vi "Number of Periods.vi"(7 "Read Value? (F)":bool, 8 "error in (no error)":errorcluster, 10 "Number of Periods (1)":u16=1 max=2000 step=1, 11 "VISA resource name":refnum<visa-resource-name>) -> (0 "error out":errorcluster, 2 "Number of Periods":u16=1, 3 "VISA resource name out":refnum<visa-resource-name>)   [LabVIEW 2013, in "SRS SR400.lvlib"]
doc: "<B>NP { m }</B>\n\nIf m is absent, the NP command returns the programmed number of periods in a scan (N PERIODS). If m is included, the number of periods is set to the value m. The parameter m must be an integer from 1 to 2000. Changing the number of periods during a scan is allowed. If the new value exceeds the current scan position, then the scan will continue to the new number of periods. If the new value is lower than the current scan position, then the scan ends at the next end of count period."
uses:
  <instrlib>/SRS SR400/SRS SR400.lvlib
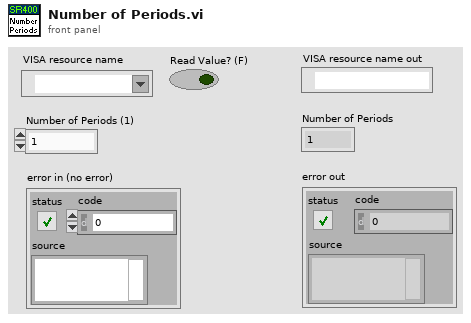
[diagram p1: front panel]
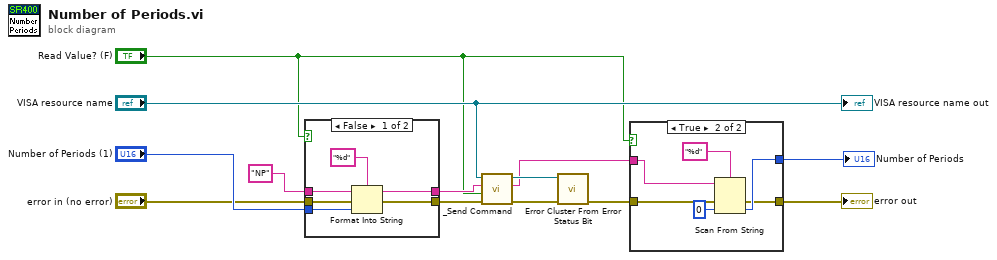
[diagram p0: block diagram]
diagram:
  n1 = case shown="False" "Read Value? (F)" {
    tunnel: "Number of Periods (1)" -> [w19 _]
    tunnel: "error in (no error)" -> [w18 w20]
    tunnel: "NP" ("command") -> [w16 w21]
    tunnel: [w15 w21] -> w10
    tunnel: [w14 w20] -> w9
    frame False {
      n2 = Format Into String(format string="%d", initial string=w16, error in=w18, w19) -> (resulting string=w15:string, error out=w14:errorcluster)
    }
    frame True {
    }
  }
  n3 = call <instrlib>:"_Send Command.vi"("error in (no error)"=w9, "Read Value? (F)"="Read Value? (F)", "Command"=w10, "VISA resource name"="VISA resource name") -> ("error out"=w6:errorcluster, "Response"=w3:string, "VISA resource name out"=w7:refnum<visa-resource-name>)  [unwired: 5 out]
  n4 = call <instrlib>:"Error Cluster From Error Status Bit.vi"("error in (no error)"=w6, "VISA resource name"=w7) -> ("error out"=w5:errorcluster)  [unwired: 8 in, 1 out]
  n5 = case shown="True" "Read Value? (F)" {
    tunnel: w5 -> [w22 w28]
    tunnel: w3 -> [_ w27]
    tunnel: [_ w24] -> w2
    tunnel: [w22 w23] -> w1
    frame False {
    }
    frame True {
      n6 = Scan From String(format string="%d", input string=w27, error in=w28, default 1=u16 0 ("default value 1")) -> (error out=w23:errorcluster, output 1=w24:u16)  [unwired: 1 in, 2 out]
    }
  }
  "error out" <- w1
  "Number of Periods" <- w2
  "VISA resource name out" <- "VISA resource name"
